vi "GetType.vi"(8 "error in (no error)":errorcluster, 11 "Configure Thermistor [THM] Msg":refnum<class "Configure Thermistor [THM] Msg.lvclass">) -> (0 "error out":errorcluster, 2 "Data Sample":variant, 3 "Configure Thermistor [THM] Msg":refnum<class "Configure Thermistor [THM] Msg.lvclass">)   [LabVIEW 2016, in "CS++DMM.lvlib" / "Configure Thermistor [THM] Msg.lvclass"]
uses:
  Configure Thermistor [THM] Msg.lvclass
  Configure Thermistor [THM] Msg.lvclass/Configure Thermistor [THM] Msg.ctl
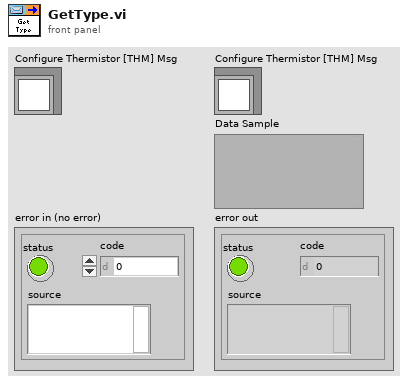
[diagram p1: front panel]
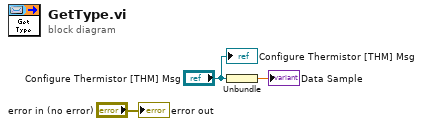
[diagram p0: block diagram]
diagram:
  n1 = Unbundle("Configure Thermistor [THM] Msg") -> (→"Data Sample":dbl)
  "error out" <- "error in (no error)"
  "Configure Thermistor [THM] Msg" <- "Configure Thermistor [THM] Msg"
